vi "Insert Into Array (Multi Boolean).vi"(9 "index":i32, 10 "Array":bool[](array[boolean]), 11 "JSON Array in":refnum<class "JSON Helper.lvclass">) -> (3 "JSON Array out":refnum<class "JSON Helper.lvclass">)   [LabVIEW 2016]
doc: "Inserts an element or subarray into a JSON array at the point you specify in index."
uses:
  JSON Helper/JSON Helper.lvclass
  JSON Boolean/New JSON Boolean.vi
  Insert Into Array (Multi).vi
  JSON Datatype/JSON Null.lvclass
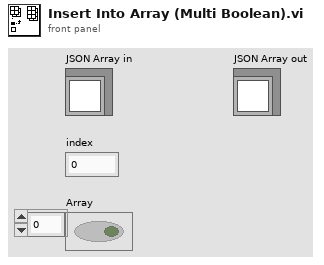
[diagram p1: front panel]
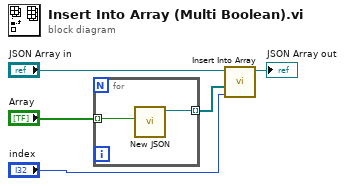
[diagram p0: block diagram]
diagram:
  n1 = for {
    tunnel: "Array" -> [w7] mode=indexing
    tunnel: [w6] -> w1 mode=indexing
    n2 = call-poly "New JSON.vi"("value"=w7) -> ("JSON Boolean out"=w6:refnum<class "JSON Helper.lvclass">)  [unwired: 9 in, 1 out]
  }
  n3 = call-poly "Insert Into Array.vi"("index"="index", "Array"=w1, "JSON Array in"="JSON Array in") -> ("JSON Array out"=→"JSON Array out":refnum<class "JSON Helper.lvclass">)  [unwired: 8 in]
